vi "CalculateSpeedOfSound.vi"(10 "Sample thickness":dbl, 11 "AScan+Peaks":cluster{"timebase":dbl[], "data":u16[]}[](array[cluster])) -> (3 "SOS":dbl[](array[numeric]))   [LabVIEW 2026]
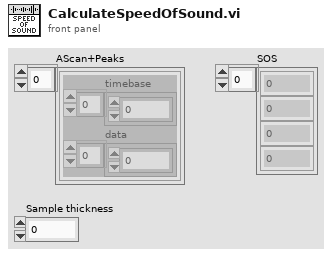
[diagram p1: front panel]
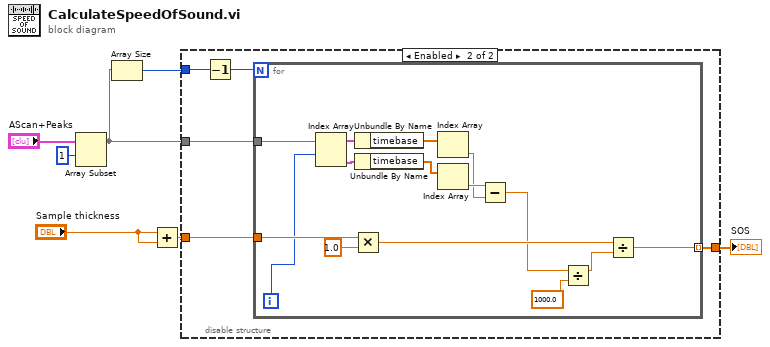
[diagram p0: block diagram]
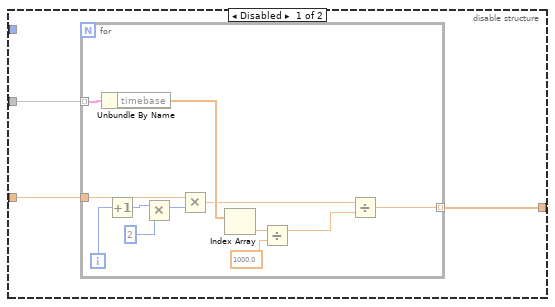
[diagram p2: hidden frame]
diagram:
  n1 = Array Subset(array="AScan+Peaks", index=1) -> (w2:cluster{"timebase":dbl[], "data":u16[]}[])  [unwired: 1 in]
  n2 = Array Size(array=w2) -> (size(s)=w1:i32)
  n3 = Add(x="Sample thickness", y="Sample thickness") -> (x+y=w6:dbl)
  n4 = disable-structure shown="Enabled" {
    disable-tunnel: w6 -> [w10 w27]
    disable-tunnel: [w9 w26] -> w5
    disable-tunnel: w2 -> [w8 w25]
    disable-tunnel: w1 -> [_ w24]
    frame Disabled {
      n5 = for {
        tunnel: w8 -> [w22] mode=indexing
        tunnel: w10 -> [w20]
        tunnel: [w18] -> w9 mode=indexing
        i -> [w14]
        n6 = Unbundle By Name(w22) -> ("timebase"=w21:dbl[])
        n7 = Increment(x=w14) -> (x+1=w13:i32)
        n8 = Multiply(x=w13, y=2 ("x")) -> (x*y=w12:i32)
        n9 = Multiply(x=w20, y=w12) -> (x*y=w15:dbl)
        n10 = Index Array(array=w21) -> (element=w19:dbl)  [unwired: 1 in]
        n11 = Divide(x=w19, y=1000.0) -> (x/y=w17:dbl)
        n12 = Divide(x=w15, y=w17) -> (x/y=w18:dbl)
      }
    }
    frame Enabled {
      n13 = Decrement(x=w24) -> (x-1=w23:i32)
      n14 = for {
        N: w23 -> [_]
        tunnel: w25 -> [w42]
        tunnel: w27 -> [w40]
        tunnel: [w39] -> w26 mode=indexing
        i -> [w28]
        n15 = Index Array(array=w42, index #1=w28) -> (element #1=w35:cluster{"timebase":dbl[], "data":u16[]}, element #2=w34:cluster{"timebase":dbl[], "data":u16[]})  [unwired: 1 in]
        n16 = Multiply(x=w40, y=1.0) -> (x*y=w36:dbl)
        n17 = Unbundle By Name(w35) -> ("timebase"=w41:dbl[])
        n18 = Unbundle By Name(w34) -> ("timebase"=w33:dbl[])
        n19 = Index Array(array=w41) -> (element=w31:dbl)  [unwired: 1 in]
        n20 = Index Array(array=w33) -> (element=w32:dbl)  [unwired: 1 in]
        n21 = Subtract(x=w32, y=w31) -> (x-y=w30:dbl)
        n22 = Divide(x=w30, y=1000.0) -> (x/y=w38:dbl)
        n23 = Divide(x=w36, y=w38) -> (x/y=w39:dbl)
      }
    }
  }
  "SOS" <- w5
